vi "Draw Rose Pointer.vi"(6 "compass pointer color":u32, 7 "draw area cache":T1, 9 "rose size (0-1)":dbl, 10 "heading (rad)":dbl, 11 "picture in":picture) -> (3 "picture out":picture)   [LabVIEW 2017, in "NI_Robotics_Compass Picture.lvlib"]
uses:
  <vilib>/robotics/Controls/Compass Indicator/Compass Picture/NI_Robotics_Compass Picture.lvlib
  <vilib>/robotics/Controls/Compass Indicator/Compass Picture/Draw Area State.ctl
  <vilib>/Utility/miscctls.llb/LVBoundsTypeDef.ctl
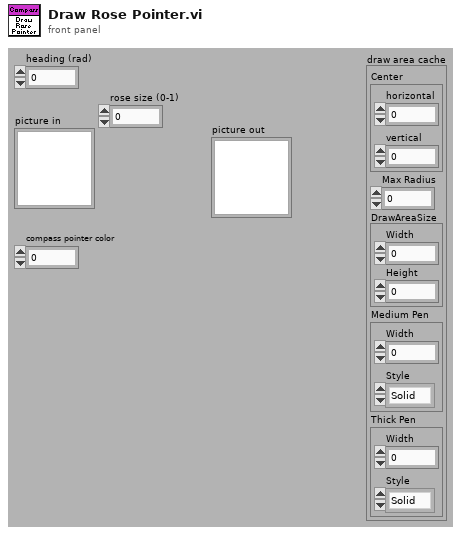
[diagram p1: front panel]
types:
  T1 = typedef "NI_Robotics_Compass Picture.lvlib/Draw Area State.ctl" = cluster{"Center":cluster{"horizontal":i16, "vertical":i16}, "Max Radius":dbl, "DrawAreaSize":T2, "Medium Pen":cluster{"Width":u16, "Style":enum32{"Solid", "Dash", "Dot", "DashDot", "DashDotDot"}}, "Thick Pen":cluster{"Width":u16, "Style":enum32{"Solid", "Dash", "Dot", "DashDot", "DashDotDot"}}}
  T2 = typedef "LVBoundsTypeDef.ctl" = cluster{"Width":u32, "Height":u32}
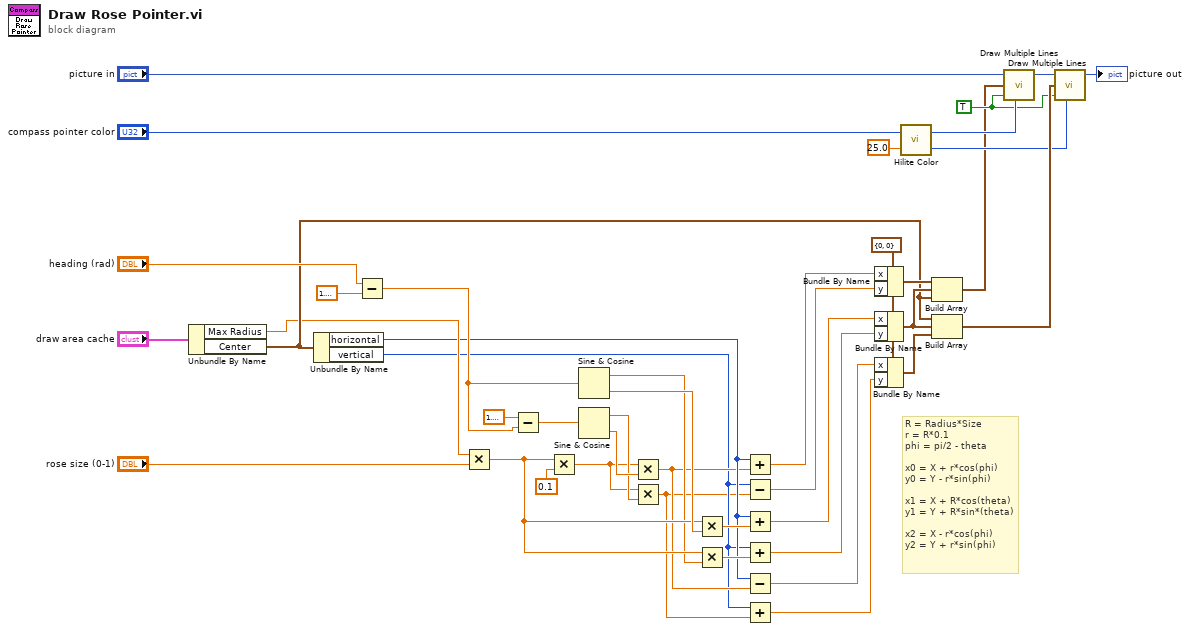
[diagram p0: block diagram]
diagram:
  w34 = TRUE ("fill?(F)")
  w29 = cluster{"x":i16, "y":i16} {"x"=0, "y"=0}
  # "R = Radius*Size\nr = R*0.1\nphi = pi/2 - theta\n\nx0 = X + r*cos(phi)\ny0 = Y - r*sin(phi)\n\nx1 = X + R*cos(theta)\ny1 = Y + R*sin*(theta)\n\nx2 = X - r*cos(phi)\ny2 = Y + r*sin(phi)"
  n1 = Unbundle By Name("draw area cache") -> ("Max Radius"=w24:dbl, "Center"=w26:cluster{"horizontal":i16, "vertical":i16})
  n2 = Unbundle By Name(w26) -> ("horizontal"=w6:i16, "vertical"=w3:i16)
  n3 = Subtract(x="heading (rad)", y=1.5707963267948966) -> (x-y=w19:dbl)
  n4 = Multiply(x=w24, y="rose size (0-1)") -> (x*y=w10:dbl)
  n5 = Subtract(x=1.5707963267948966, y=w19) -> (x-y=w20:dbl)
  n6 = Multiply(x=w10, y=0.1) -> (x*y=w14:dbl)
  n7 = Sine & Cosine(0:w19) -> (1:w9:dbl, 2:w13:dbl)
  n8 = Sine & Cosine(0:w20) -> (1:w16:dbl, 2:w18:dbl)
  n9 = Multiply(x=w14, y=w18) -> (x*y=w5:dbl)
  n10 = Multiply(x=w14, y=w16) -> (x*y=w2:dbl)
  n11 = Multiply(x=w10, y=w13) -> (x*y=w12:dbl)
  n12 = Multiply(x=w10, y=w9) -> (x*y=w8:dbl)
  n13 = Add(x=w6, y=w5) -> (x+y=w17:dbl)
  n14 = Subtract(x=w3, y=w2) -> (x-y=w15:dbl)
  n15 = Add(x=w6, y=w12) -> (x+y=w11:dbl)
  n16 = Add(x=w3, y=w8) -> (x+y=w7:dbl)
  n17 = Subtract(x=w6, y=w5) -> (x-y=w4:dbl)
  n18 = Add(x=w3, y=w2) -> (x+y=w1:dbl)
  n19 = Bundle By Name(cluster=w29, "x"=w17, "y"=w15) -> (w30:cluster{"x":i16, "y":i16})
  n20 = Bundle By Name(cluster=w29, "x"=w11, "y"=w7) -> (w38:cluster{"x":i16, "y":i16})
  n21 = Bundle By Name(cluster=w29, "x"=w4, "y"=w1) -> (w37:cluster{"x":i16, "y":i16})
  n22 = call <vilib>:"Hilite Color.vi"("Percentage(30)"=25.0, "Color In"="compass pointer color") -> ("Shadow"=w40:u32, "Hilite"=w39:u32)
  n23 = Build Array(w30, w38, w26) -> (w31:cluster{"horizontal":i16, "vertical":i16}[])
  n24 = Build Array(w26, w38, w37) -> (w41:cluster{"x":i16, "y":i16}[])
  n25 = call <vilib>:"Draw Multiple Lines.vi"("picture"="picture in", "line endpoints"=w31, "fill?(F)"=w34, "color(black)"=w39) -> ("new picture"=w35:picture)  [unwired: 5 in]
  n26 = call <vilib>:"Draw Multiple Lines.vi"("picture"=w35, "line endpoints"=w41, "fill?(F)"=w34, "color(black)"=w40) -> ("new picture"=→"picture out":picture)  [unwired: 5 in]
